vi "Thread@ForeachStart__Parameter.vi"(1 "ParamterIn":string) -> (0 "ParamterOut":string)   [LabVIEW 2019]
panel:
  in  "Thread Label":string(combo)
  in  "Confirm":bool
  # "Thread@ForeachStart $Label"
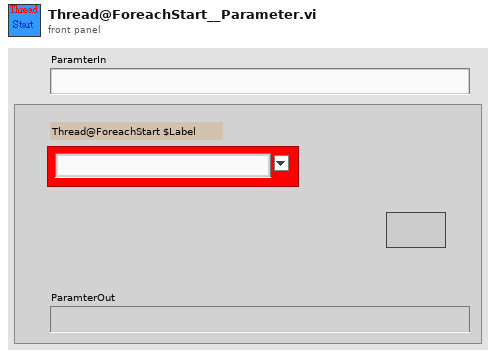
[diagram p1: front panel]
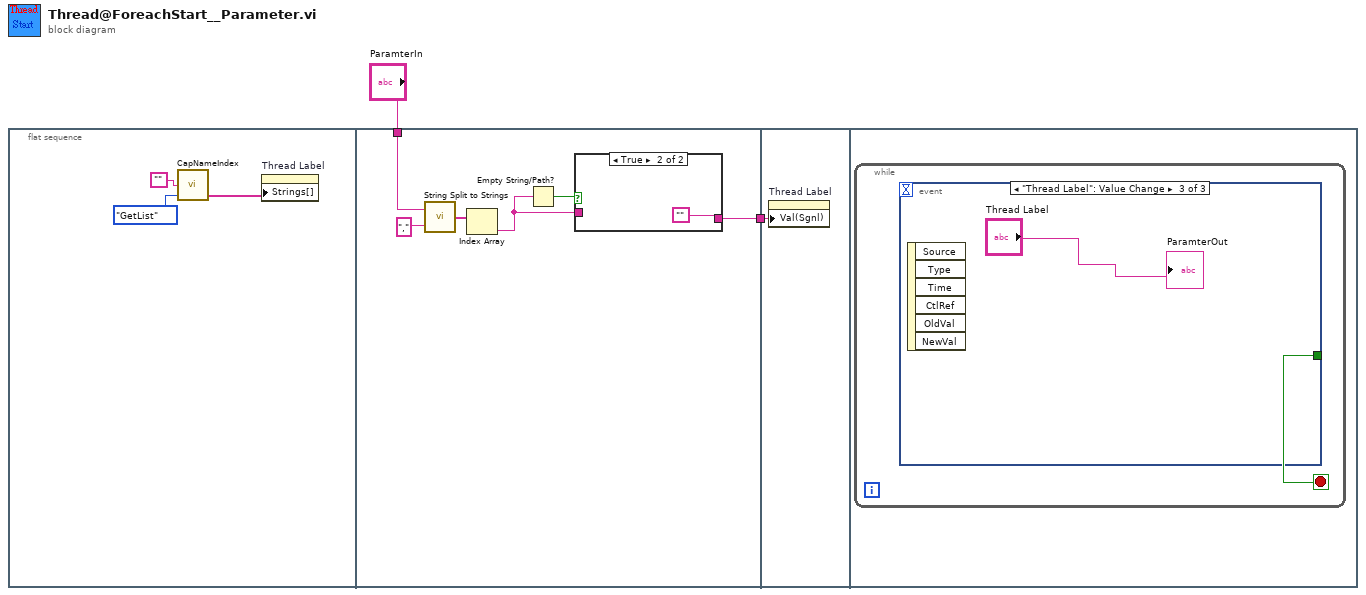
[diagram p0: block diagram]
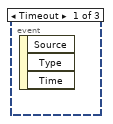
[diagram p3: hidden frame]
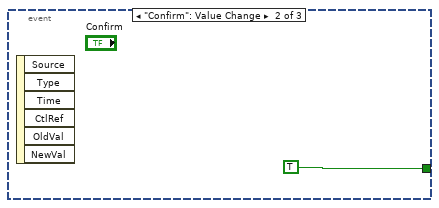
[diagram p4: hidden frame]
diagram:
  n1 = flat-sequence {
    tunnel: "ParamterIn" -> [w9]
    tunnel: [w6] -> w1
    tunnel: w1 -> [w14]
    frame #0 {
      n2 = call "CapNameIndex.vi"("OP"=enum16{"AddCam", "GetIndex", "Init", "GetList"}."GetList", "CamName"="") -> ("DeviceList"=w4:string[])  [unwired: 1 in, 2 out]
      n3 = property on="Thread Label" class="CmbBox"("Strings[]"=w4) -> ()  [unwired: 2 in, 2 out]
    }
    frame #1 {
      n4 = call "String Split to Strings.vi"("search string/char (-)"=",", "String"=w9) -> ("Array"=w11:string[])
      n5 = Index Array(array=w11) -> (element=w7:string)  [unwired: 1 in]
      n6 = Empty String/Path?(string/path=w7) -> (empty?=w8:bool)
      n7 = case shown="True" w8 {
        tunnel: w7 -> [w12 _]
        tunnel: [w12 ""] -> w6
        frame False {
        }
        frame True {
        }
      }
    }
    frame #2 {
      n8 = property on="Thread Label" class="CmbBox"("Val(Sgnl)"=w14) -> ()  [unwired: 2 in, 2 out]
    }
    frame #3 {
      n9 = while {
        stop <- w15 stop-if-true
        n10 = event shown="[2] \"Thread Label\": Value Change" {
          selector: _ -> [_ _ _]
          dyn-events: _ -> [_ _ _]
          timeout: _ -> [_ _ _]
          tunnel: [_ TRUE _] -> w15
          event Timeout {
            n11 = event-data() -> ()  [unwired: 1 in, 3 out]
          }
          event "Confirm": Value Change {
            n12 = event-data() -> ()  [unwired: 1 in, 6 out]
          }
          event "Thread Label": Value Change {
            n13 = event-data() -> ()  [unwired: 1 in, 6 out]
            "ParamterOut" <- "Thread Label"
          }
        }
      }
    }
  }
